vi "Control_Relays.vi"(7 "Test_Configuration":enum16{"Throws", "Guardian"}(ring), 8 "Error In":errorcluster, 11 "instrument handle":refnum<k15>) -> (0 "Error Out":errorcluster)   [LabVIEW 2013]
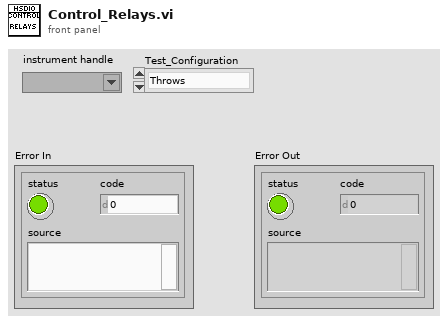
[diagram p1: front panel]
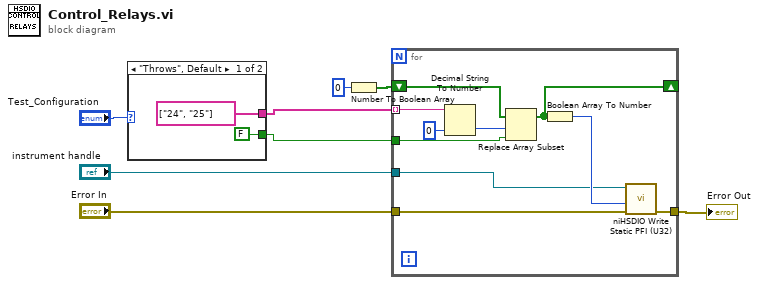
[diagram p0: block diagram]
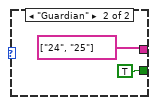
[diagram p2: hidden frame]
diagram:
  n1 = case shown="\"Throws\", Default" "Test_Configuration" {
    tunnel: [string[] ["24", "25"] string[] ["24", "25"]] -> w5
    tunnel: [FALSE ("Boolean") TRUE ("Boolean")] -> w4
    frame "Throws", Default {
    }
    frame "Guardian" {
    }
  }
  n2 = Number To Boolean Array(number=0 ("Numeric")) -> (Boolean array=w7:bool[])
  n3 = for {
    shift-right: [w19] -> _
    shift-left: w7 -> [w20]
    tunnel: w5 -> [w17] mode=indexing
    tunnel: "Error In" -> [w16]
    tunnel: [w15] -> w1
    tunnel: "instrument handle" -> [w14]
    tunnel: w4 -> [w13]
    n4 = Decimal String To Number(string=w17, default (0L)=0 ("default (0 I32)")) -> (number=w21:i32)  [unwired: 1 in, 1 out]
    n5 = Replace Array Subset(array=w20, new element=w13, index=w21) -> (w19:bool[])
    n6 = Boolean Array To Number(Boolean array=w19) -> (number=w18:u32)
    n7 = call <instrlib>:"niHSDIO Write Static PFI (U32).vi"("error in (no error)"=w16, "channel mask (no masking:-1)"=w18, "instrument handle"=w14) -> ("error out"=w15:errorcluster)  [unwired: 7 in, 1 out]
  }
  "Error Out" <- w1
